vi "MRC Alert Create Alert.vi"(7 "level":i32, 8 "error in (no error)":errorcluster, 9 "text":T1, 10 "uniqueId":T1, 11 "group":T1) -> (0 "error out":errorcluster, 3 "handle out":i64)   [LabVIEW 2026, in "MrcLib.lvlib"]
doc: "MRC_Status MRC_CALLCONV MRC_Alert_CreateAlert(const struct MRC_String* group,\n const struct MRC_String* uniqueId,\n const struct MRC_String* text,\n int32_t level,\n MRC_AlertHandle* handle);"
uses:
  MrcLib.lvlib
  <vilib>/MRC/Types/MRC String.ctl
  MrcLib.dll
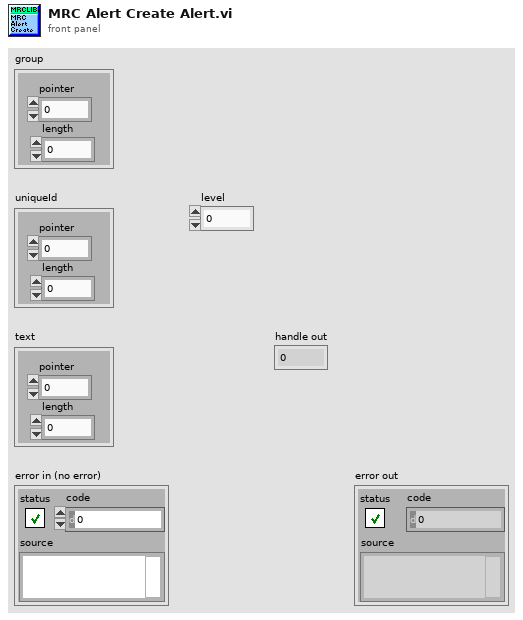
[diagram p1: front panel]
types:
  T1 = typedef "MRC String.ctl" = cluster{"pointer":u64, "length":u64}
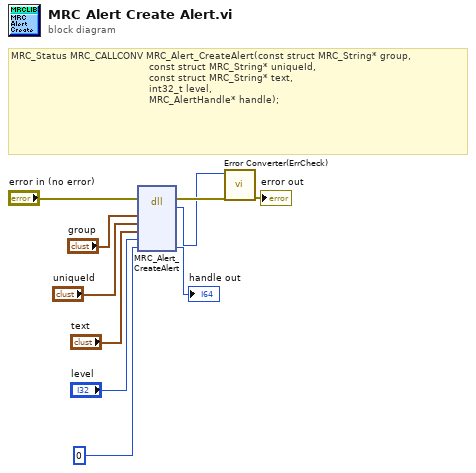
[diagram p0: block diagram]
diagram:
  # "MRC_Status MRC_CALLCONV MRC_Alert_CreateAlert(const struct MRC_String* group,\n                                              const struct MRC_String* uniqueId,\n                                              const struct MRC_String* text,\n                                              int32_t level,\n                                              MRC_AlertHandle* handle);"
  n1 = dll-call lib="MrcLib.*" fn="MRC_Alert_CreateAlert"(error in="error in (no error)", "group"="group", "uniqueId"="uniqueId", "text"="text", "level"="level", "handle"=i64 0) -> (error out=w3:errorcluster, "return type"=w1:i32, "handle"=→"handle out":i64)  [unwired: 6 in, 1 out]
  n2 = call <vilib>:"Error Converter(ErrCheck).vi"("error in (no error)"=w3, "status"=w1) -> ("error out"=→"error out":errorcluster)  [unwired: 9 in]
